vi "CH_LM App Interface Dialog.vi"() -> ()   [LabVIEW 2012, in "CH_LM App.lvlib"]
doc: "This VI is a dialog to ask the user for the meter addresses to use."
uses:
  CH_LM App.lvlib
  CH_LM/CH_LM Communication Mode.ctl
  CH_LM.lvlib
  CH_LM/CH_LM BaudRates.ctl
  CH_LM/CH_LM Parity.ctl
  CH_LM/CH_LM SerialConfiguration.ctl
  CH_LM App Connection Info.ctl
panel:
  out "Address":i32
  in  "Connection Info":T1={"Address"=1, "Serial Configuration\n(19200,N,8,1)"={"Baud Rate"=19200, "Parity"=0, "Data Bits"=8, "Stop Bits"=1}} {"Serial Configuration\n(19200,N,8,1)"."Parity" items=["None", "Odd", "Even"]; "Serial Configuration\n(19200,N,8,1)"."Baud Rate" items=["9600"=9600, "19200"=19200, "38400"=38400, "57600"=57600, "115200"=115200]}
  out "Communication Mode":T5=enum."USB"
  in  "Connection Info":T1[](array[typedef]) {"Serial Configuration\n(19200,N,8,1)"."Parity" items=["None", "Odd", "Even"]; "Serial Configuration\n(19200,N,8,1)"."Baud Rate" items=["9600"=9600, "19200"=19200, "38400"=38400, "57600"=57600, "115200"=115200]}
  in  "Cancel":bool
  in  "Connect?":bool
  # "Add element\nfor each\nLabMax to use"
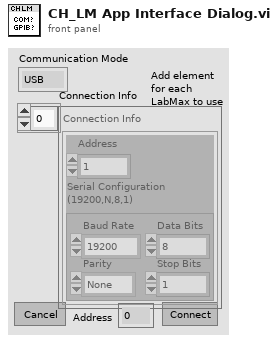
[diagram p1: front panel]
types:
  T1 = typedef "CH_LM App.lvlib/CH_LM App Connection Info.ctl" = cluster{"Address":i32, "Serial Configuration\n(19200,N,8,1)":T2}
  T2 = typedef "CH_LM.lvlib/CH_LM SerialConfiguration.ctl" = cluster{"Baud Rate":T3, "Parity":T4, "Data Bits":u16, "Stop Bits":u16}
  T3 = typedef "CH_LM.lvlib/CH_LM BaudRates.ctl" = u32
  T4 = typedef "CH_LM.lvlib/CH_LM Parity.ctl" = u16
  T5 = typedef "CH_LM.lvlib/CH_LM Communication Mode.ctl" = enum16{"None", "USB", "GPIB", "RS232"}
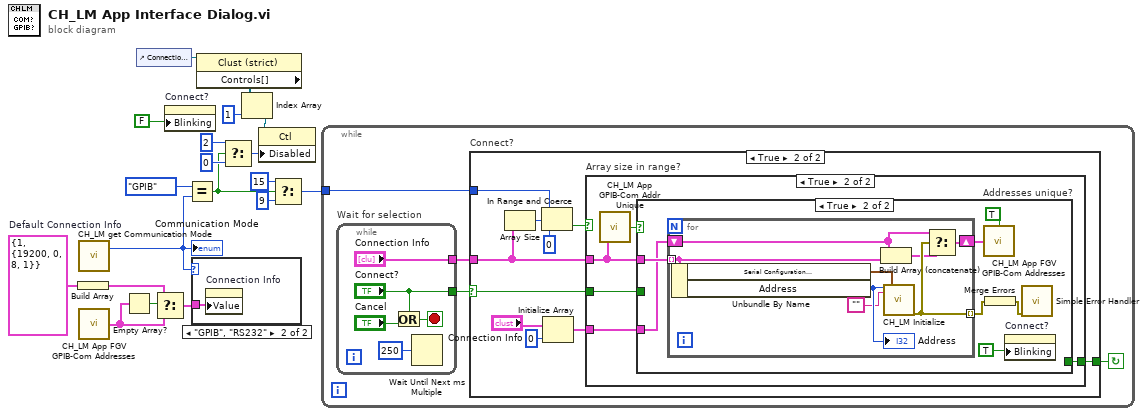
[diagram p0: block diagram]
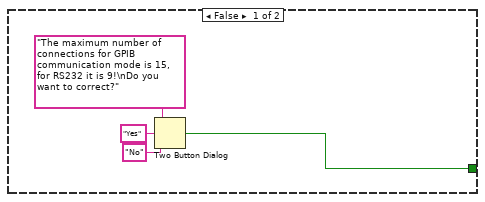
[diagram p4: hidden frame]
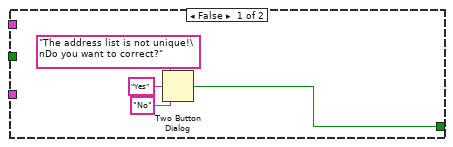
[diagram p5: hidden frame]
diagram:
  w2 = T1 {"Address"=1, "Serial Configuration\n(19200,N,8,1)"={"Baud Rate"=19200, "Parity"=0, "Data Bits"=8, "Stop Bits"=1}}  # Default Connection Info
  n1 = Build Array(w2) -> (w1:T1[])
  n2 = call "CH_LM get Communication Mode.vi"() -> ("Communication Mode"=w6:T5)  [unwired: 1 in, 2 out]
  "Communication Mode" <- w6
  n3 = call "CH_LM App FGV GPIB-Com Addresses.vi"() -> ("Connection Array"=w4:T1[])  [unwired: 2 in]
  n4 = Empty Array?(array=w4) -> (empty?=w5:bool)
  n5 = control-ref of="Connection Info"() -> (w15:refnum<vi>)
  n6 = Select(t=w1, s=w5, f=w4) -> (s? t:f=w3:T1[])
  n7 = property on="Connect?" class="Bool"("Blinking"=FALSE) -> ()  [unwired: 2 in, 2 out]
  n8 = Equal?(x=CH_LM_Communication_Mode."GPIB" ("Communication Mode"), y=w6) -> (x = y?=w9:bool)
  n9 = case shown="\"GPIB\", \"RS232\"" w6 {
    tunnel: w3 -> [_ w20]
    frame Default {
    }
    frame "GPIB", "RS232" {
      n10 = property on="Connection Info" class="Arr (strict)"("Value"=w20) -> ()  [unwired: 2 in, 2 out]
    }
  }
  n11 = property class="Clust (strict)"(reference=w15) -> ("Controls[]"=w14:refnum<vi>[])  [unwired: 1 in, 2 out]
  n12 = Select(t=u8 2 ("Disabled"), s=w9, f=u8 0 ("Disabled")) -> (s? t:f=w8:u8)
  n13 = Index Array(array=w14, index=1) -> (element=w12:refnum<vi>)
  n14 = property class="Ctl"(reference=w12, "Disabled"=w8) -> ()  [unwired: 1 in, 2 out]
  n15 = Select(t=15 ("lower limit"), s=w9, f=9) -> (s? t:f=w16:i32)
  n16 = while {
    tunnel: w16 -> [w22]
    stop <- w24 continue-if-true
    n17 = while "Wait for selection" {
      tunnel: ["Connection Info"] -> w23
      tunnel: ["Connect?"] -> w21
      stop <- w68 stop-if-true
      n18 = Or(x="Connect?", y="Cancel") -> (x .or. y?=w68:bool)
      n19 = Wait Until Next ms Multiple(millisecond multiple=u32 250) -> ()  [unwired: 1 out]
    }
    n20 = case "Connect?" shown="True" w21 {
      selector: w21 -> [w25 w26]
      tunnel: [w25 w35] -> w24
      tunnel: w23 -> [_ w34]
      tunnel: w22 -> [_ w31]
      frame False {
      }
      frame True {
        n21 = Array Size(array=w34) -> (size(s)=w33:i32)
        n22 = In Range and Coerce(upper limit=w31, x=w33, lower limit=0) -> (In Range?=w30:bool)  [unwired: 1 out]
        n23 = Initialize Array("Connection Info", 0 ("dimension size")) -> (w27:T1[])
        n24 = case "Array size in range?" shown="True" w30 {
          tunnel: w26 -> [_ w44]
          tunnel: [w36 w42] -> w35
          tunnel: w34 -> [_ w41]
          tunnel: w27 -> [_ w40]
          frame False {
            n25 = Two Button Dialog(message="The maximum number of connections for GPIB communication mode is 15, for RS232 it is 9!\nDo you want to correct?", 1:"No" ("F button name (\"Cancel\")"), 2:"Yes" ("T button name (\"OK\")")) -> (T button?=w36:bool)
          }
          frame True {
            n26 = call "CH_LM App GPIB-Com Addr Unique.vi"("Address Array"=w41) -> ("Unique?"=w43:bool)
            n27 = case "Addresses unique?" shown="True" w43 {
              tunnel: w44 -> [_ _]
              tunnel: w41 -> [_ w55]
              tunnel: [w45 _] -> w42
              tunnel: w40 -> [_ w51]
              frame False {
                n28 = Two Button Dialog(message="The address list is not unique!\nDo you want to correct?", 1:"No" ("F button name (\"Cancel\")"), 2:"Yes" ("T button name (\"OK\")")) -> (T button?=w45:bool)
              }
              frame True {
                n29 = for {
                  tunnel: w55 -> [w59] mode=indexing
                  tunnel: [w62] -> w54 mode=indexing
                  shift-right: [w61] -> w50
                  shift-left: w51 -> [w60]
                  n30 = Unbundle By Name(w59) -> ("Serial Configuration\n(19200,N,8,1)"=w63:T2, "Address"=w57:i32)
                  "Address" <- w57
                  n31 = Build Array (concatenate)(w60, w59) -> (w58:T1[])
                  n32 = call "CH_LM Initialize.vi"("Address"=w57, "Serial Number"="", "Serial Configuration\n(19200,N,8,1)"=w63) -> ("error out"=w62:errorcluster)  [unwired: 2 in, 14 out]
                  n33 = Select(t=w60, s=w62, f=w58) -> (s? t:f=w61:T1[])
                }
                n34 = call "CH_LM App FGV GPIB-Com Addresses.vi"("Connection Array"=w50, "set? (F)"=TRUE) -> ()  [unwired: 1 out]
                n35 = Merge Errors(w54) -> (w53:errorcluster)
                n36 = property on="Connect?" class="Bool"("Blinking"=TRUE) -> ()  [unwired: 2 in, 2 out]
                n37 = call <vilib>:"Simple Error Handler.vi"("error in (no error)"=w53) -> ()  [unwired: 1 in, 8 out]
              }
            }
          }
        }
      }
    }
  }
